vi "SetExposureTime.vi"(0 "Time":sgl=-inf format="%#_g µs", 5 "error in":T1) -> (14 "Time out":sgl format="%#_g µs", 19 "error out":T1)   [LabVIEW 2016]
doc: "This VI sets the exposure time in us. By passing -Inf (float) as input values, the current exposure time will be read out."
uses:
  Controls/Error_Out.ctl
  Files_ASC500/DLL/ASC500_RemoteControlV27.dll
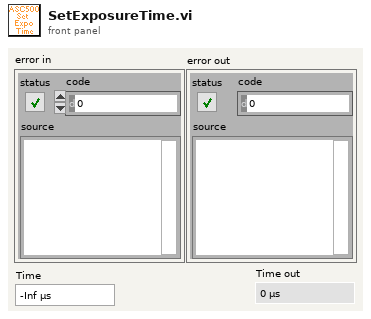
[diagram p1: front panel]
types:
  T1 = typedef "Error_Out.ctl" = errorcluster
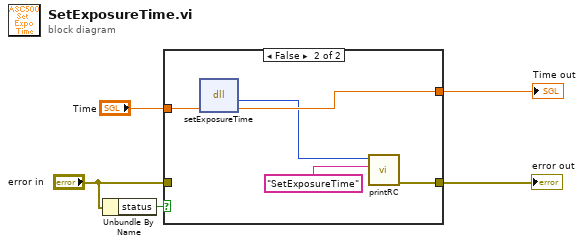
[diagram p0: block diagram]
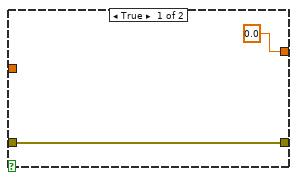
[diagram p2: hidden frame]
diagram:
  n1 = Unbundle By Name("error in") -> ("status"=w5:bool)
  n2 = case shown="False" w5 {
    tunnel: [w6 w10] -> w4
    tunnel: "Time" -> [_ w12]
    tunnel: [sgl 0.0 ("Time") w11] -> w2
    tunnel: "error in" -> [w6 _]
    frame True {
    }
    frame False {
      n3 = dll-call lib="G:/SCMOperations/Share/ELE/Produkt Information/ASC500/04 Remote Control/02 development versions/2018Nov06/Files_ASC500/DLL/ASC500_RemoteControlV27.dll" fn="setExposureTime"("Time"=w12) -> ("return type"=w9:i32, "Time"=w11:sgl)  [unwired: 3 in, 2 out]
      n4 = call "printRC.vi"("additional information"="SetExposureTime", "RC"=w9) -> ("error out"=w10:T1)  [unwired: 9 in]
    }
  }
  "error out" <- w4
  "Time out" <- w2
